vi "Robot Global Data.vi"() -> ()   [LabVIEW 2014]
doc: "This global VI can contain as many global variables as you need. Place a control on the panel, give it a good name. To read or write to it from a VI, drag the icon to the diagram of that VI. You can also drag from the project. Click on the node to change which global you access. You shouldn't have multiple locations writing to a global or it will cause a race-condition."
uses:
  <vilib>/Rock Robotics/WPI/Camera/WPI_CameraImageSize.ctl
  <vilib>/Rock Robotics/WPI/DriverStation/WPI_DriverStationRobotMode2.ctl
  2014 Vision Dashboard Test/TargetType.ctl
panel:
  in  "goto setting 2":bool
  in  "goto setting 1":bool
  in  "Pot Max":dbl
  in  "Pot Min":dbl
  out "Autonomous Trigger":bool
  in  "Claw Rev speed":dbl
  in  "ClawFlw speed":dbl
  in  "Wait For Retract":dbl
  in  "Wait For Extend":dbl
  in  "Wait Brake Up":dbl
  in  "Wait Brake Down":dbl
  in  "Window Motor Speed":dbl
  in  "Potentiometer Zero Value":dbl
  out "Hot Target":bool
  out "Distances":T2(array[cluster])
  in  "Robot Mode":T3
  in  "LED toggle rate (ms)":u32=20
  in  "image size":T4=enum."320x240"
  in  "Enable Vision":bool
  # "INI Values"
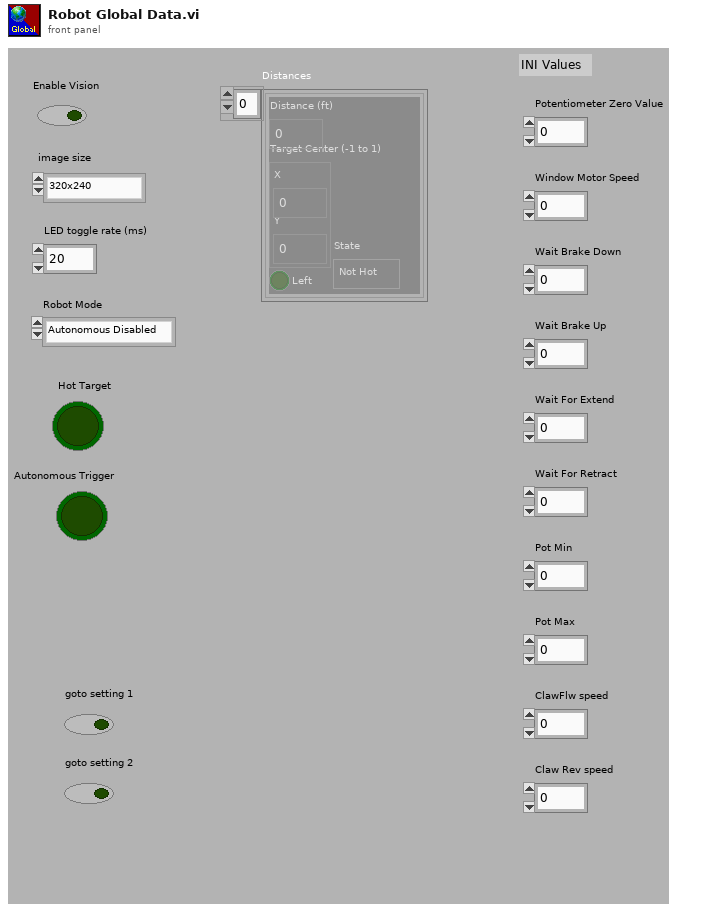
[diagram p1: front panel]
types:
  T1 = typedef "TargetType.ctl" = enum16{"Not Hot", "Hot"}
  T2 = cluster{"Distance (ft)":dbl, "Target Center (-1 to 1)":cluster{"X":dbl, "Y":dbl}, "Left":bool, "State":T1}[]
  T3 = typedef "WPI_DriverStationRobotMode2.ctl" = enum16{"Autonomous Disabled", "Autonomous Enabled", "Teleop Disabled", "Teleop Enabled", "Disconnected", "Finish", "Test Disabled", "Test Enabled", "Emergency Stopped"}
  T4 = typedef "WPI_CameraImageSize.ctl" = enum16{"640x480", "320x240", "160x120", "Custom"}
diagram:
